vi "XY Graph Invert Plots Selection Event.vi"(8 "Error In":errorcluster, 11 "XYGraph Ref":T1) -> (0 "Error Out":errorcluster, 1 "Message":string, 3 "XYGraph Ref":T1, 5 "Graph Caption":string)   [LabVIEW 2019, in "XY Graph Add-Ons.lvlib"]
uses:
  XY Graph Add-Ons.lvlib
  XY Graph Refnum.ctl
  <vilib>/Utility/High Resolution Relative Seconds.vi
panel:
  out "CPU (s)":dbl
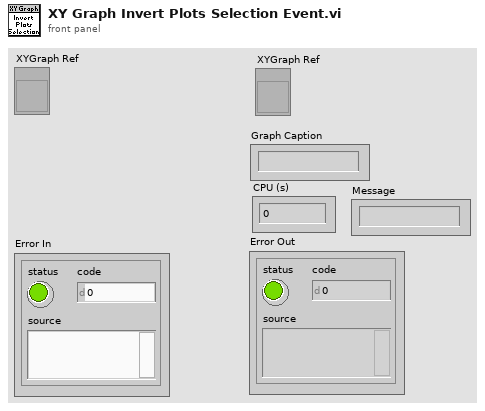
[diagram p1: front panel]
types:
  T1 = typedef "XY Graph Add-Ons.lvlib/XY Graph Refnum.ctl" = refnum<vi>
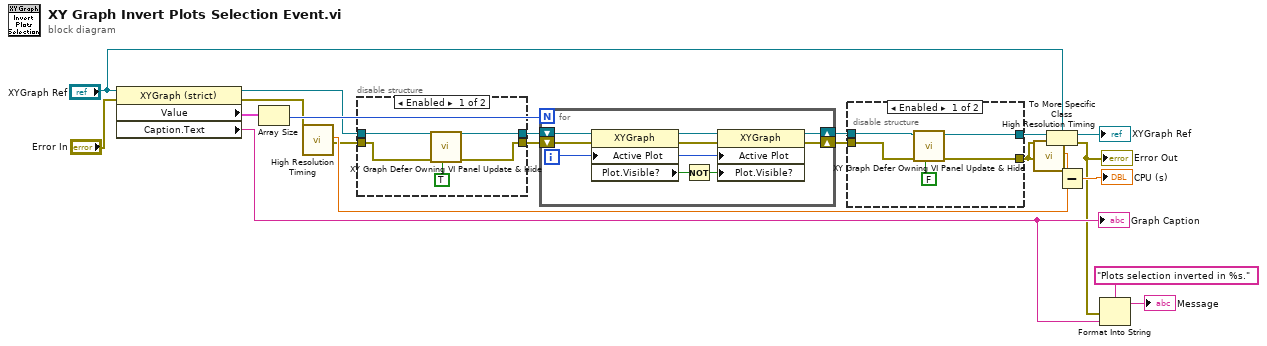
[diagram p0: block diagram]
diagram:
  n1 = property class="XYGraph (strict)"(reference="XYGraph Ref", error in="Error In") -> (reference out=w19:T1, error out=w18:errorcluster, "Value"=w21:cluster{"X Array":dbl[], "Y Array":dbl[]}[], "Caption.Text"=w3:string)
  "Graph Caption" <- w3
  n2 = Array Size(array=w21) -> (size(s)=w20:i32)
  n3 = call "High Resolution Timing.vi"("Error In"=w18) -> ("elapsed (relative) seconds"=w15:dbl, "Error Out"=w12:errorcluster)  [unwired: 16 in, 1 out]
  n4 = disable-structure shown="Enabled" {
    disable-tunnel: w19 -> [w26 w28]
    disable-tunnel: [w25 w28] -> w13
    disable-tunnel: w12 -> [w24 w27]
    disable-tunnel: [w23 w27] -> w11
    frame Enabled {
      n5 = call "XY Graph Defer Owning VI Panel Update & Hide.vi"("Defer Owning Panel Update"=TRUE ("Hide (F)/Show (T) Graph"), "error in (no error)"=w24, "XY Graph Refnum in"=w26) -> ("error out"=w23:errorcluster, "XY Graph Refnum out"=w25:refnum<vi>)  [unwired: 7 in]
    }
    frame Disabled {
    }
  }
  n6 = for {
    N: w20 -> [_]
    shift-right: [w33] -> w10
    shift-left: w13 -> [w37]
    shift-right: [w32] -> w9
    shift-left: w11 -> [w36]
    i -> [w31]
    n7 = property class="XYGraph"(reference=w37, error in=w36, "Active Plot"=w31) -> (reference out=w35:refnum<vi>, error out=w34:errorcluster, "Plot.Visible?"=w30:bool)
    n8 = Not(x=w30) -> (.not. x?=w29:bool)
    n9 = property class="XYGraph"(reference=w35, error in=w34, "Active Plot"=w31, "Plot.Visible?"=w29) -> (reference out=w33:refnum<vi>, error out=w32:errorcluster)
  }
  n10 = disable-structure shown="Enabled" {
    disable-tunnel: w10 -> [w42 _]
    disable-tunnel: w9 -> [w41 w43]
    disable-tunnel: [w40 w43] -> w5
    disable-tunnel: [w38 _] -> w8
    frame Enabled {
      n11 = call "XY Graph Defer Owning VI Panel Update & Hide.vi"("Defer Owning Panel Update"=FALSE ("Hide (F)/Show (T) Graph"), "error in (no error)"=w41, "XY Graph Refnum in"=w42) -> ("error out"=w40:errorcluster, "XY Graph Refnum out"=w38:refnum<vi>)  [unwired: 7 in]
    }
    frame Disabled {
    }
  }
  n12 = call "High Resolution Timing.vi"("Error In"=w5) -> ("elapsed (relative) seconds"=w16:dbl)  [unwired: 16 in, 2 out]
  n13 = To More Specific Class(target class="XYGraph Ref", reference=w8, error in=w5) -> (specific class reference=→"XYGraph Ref":T1, error out=w1:errorcluster)
  "Error Out" <- w1
  n14 = Subtract(x=w16, y=w15) -> (x-y=→"CPU (s)":dbl)
  n15 = Format Into String(format string="Plots selection inverted in %s.", error in=w1, w3) -> (resulting string=→"Message":string)  [unwired: 1 in, 1 out]
